vi "QuickDrop Toggle breakpoint.vi"(6 "Variant in":variant, 7 "Shift Pressed?":bool, 8 "error in (no error)":errorcluster, 10 "QD Combo Box Ref":refnum<vi>, 11 "QD Launch VI Ref":refnum<vi>) -> (0 "error out":errorcluster, 4 "Variant out":variant)   [LabVIEW 2022 SP3]
doc: "<b>Quick drop box tool:</b> Toggles breakpoints on the selected wires\n\nDefault Shortcut - [B]"
uses:
  <vilib>/Utility/miscctls.llb/LVBreakpointStatusEnum.ctl
panel:
  in  "Undo Name":string="Create Inputs and/or Outputs"
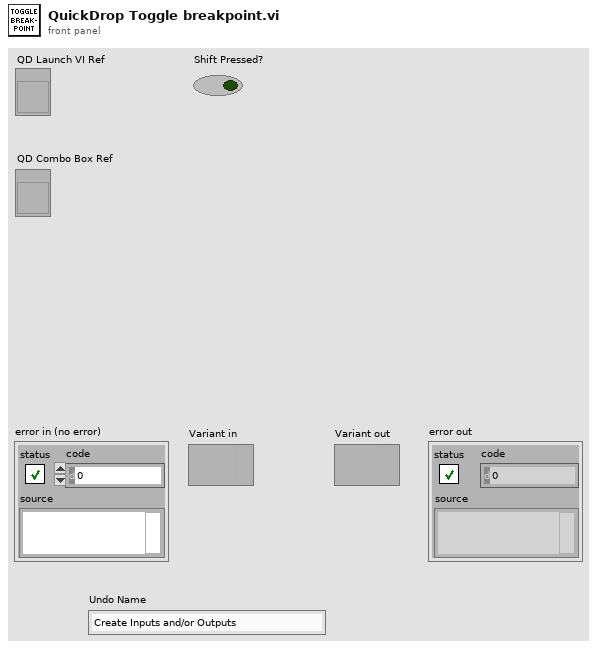
[diagram p1: front panel]
types:
  T1 = typedef "LVBreakpointStatusEnum.ctl" = enum8{"Cleared Break", "Enabled Break", "Disabled Break"}
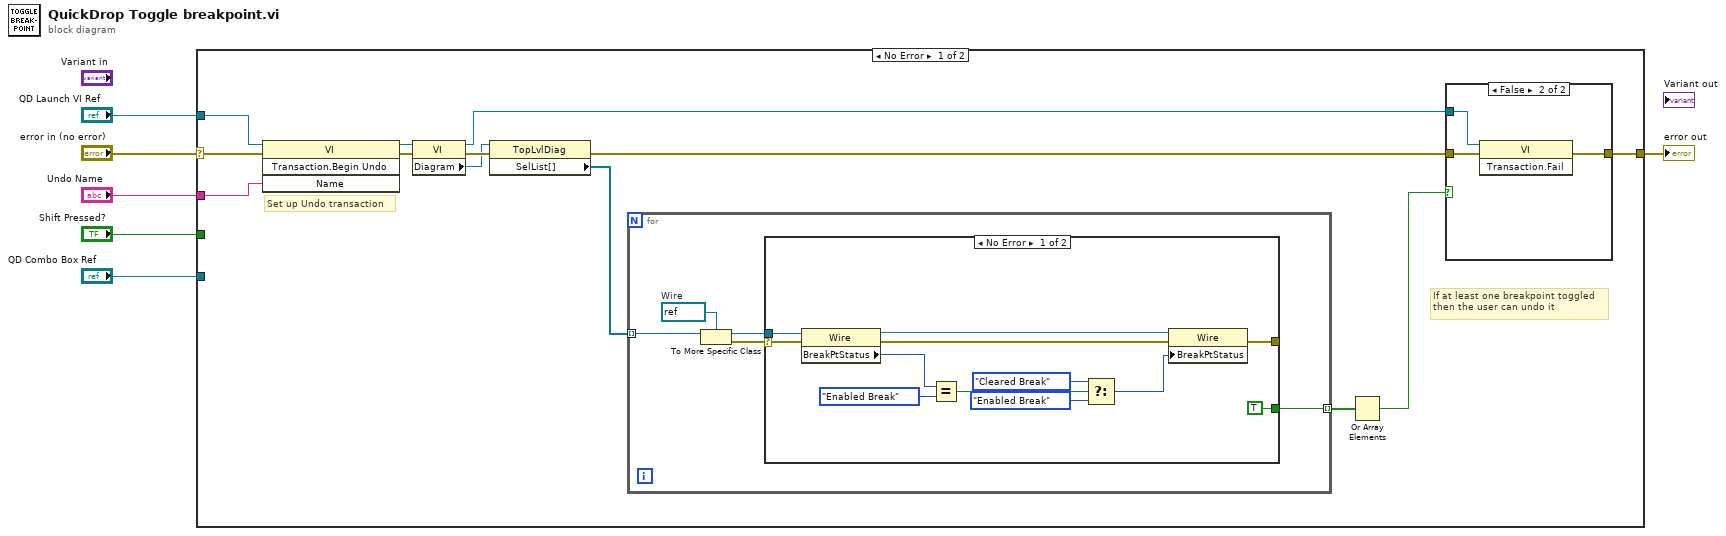
[diagram p0: block diagram]
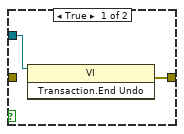
[diagram p2: hidden frame]
diagram:
  n1 = case shown="No Error" "error in (no error)" {
    selector: "error in (no error)" -> [w19 w42]
    tunnel: [w14 w42] -> w5
    tunnel: "Shift Pressed?" -> [_ _]
    tunnel: "QD Combo Box Ref" -> [_ _]
    tunnel: "QD Launch VI Ref" -> [w9 _]
    tunnel: "Undo Name" -> [w13 _]
    frame No Error {
      # "If at least one breakpoint toggled\nthen the user can undo it"
      # "Set up Undo transaction"
      n2 = invoke class="VI" method="Transaction.Begin Undo"(reference=w9, error in=w19, "Name"=w13) -> (reference out=w15:refnum<vi>, error out=w16:errorcluster)  [unwired: 1 in, 2 out]
      n3 = property class="VI"(reference=w15, error in=w16) -> (reference out=w12:refnum<vi>, error out=w18:errorcluster, "Diagram"=w17:refnum<vi>)
      n4 = property class="TopLvlDiag"(reference=w17, error in=w18) -> (error out=w7:errorcluster, "SelList[]"=w11:refnum<vi>[])  [unwired: 1 out]
      n5 = for {
        tunnel: w11 -> [w25] mode=indexing
        tunnel: [w29] -> w10 mode=indexing
        w28 = refnum<vi> refnum  # Wire
        n6 = To More Specific Class(target class=w28, reference=w25) -> (specific class reference=w26:refnum<vi>, error out=w27:errorcluster)  [unwired: 1 in]
        n7 = case shown="No Error" w27 {
          selector: w27 -> [w38 _]
          tunnel: [TRUE _] -> w29
          tunnel: w26 -> [w30 _]
          tunnel: [w31 _] -> _
          frame No Error {
            n8 = property class="Wire"(reference=w30, error in=w38) -> (reference out=w32:refnum<vi>, error out=w37:errorcluster, "BreakPtStatus"=w40:T1)
            n9 = Equal?(x=w40, y=LVBreakpointStatusEnum."Enabled Break") -> (x = y?=w36:bool)
            n10 = Select(t=LVBreakpointStatusEnum."Cleared Break", s=w36, f=LVBreakpointStatusEnum."Enabled Break") -> (s? t:f=w33:T1)
            n11 = property class="Wire"(reference=w32, error in=w37, "BreakPtStatus"=w33) -> (error out=w31:errorcluster)  [unwired: 1 out]
          }
          frame Error {
          }
        }
      }
      n12 = Or Array Elements(Boolean array=w10) -> (logical OR=w8:bool)
      n13 = case shown="False" w8 {
        tunnel: w12 -> [w20 w23]
        tunnel: [w21 w24] -> w14
        tunnel: w7 -> [_ w22]
        frame True {
          n14 = invoke class="VI" method="Transaction.End Undo"(reference=w20) -> (error out=w21:errorcluster)  [unwired: 2 in, 2 out]
        }
        frame False {
          n15 = invoke class="VI" method="Transaction.Fail"(reference=w23, error in=w22) -> (error out=w24:errorcluster)  [unwired: 1 in, 2 out]
        }
      }
    }
    frame Error {
    }
  }
  "error out" <- w5
